vi "test_Variant to KVP.vi"(8 "error in (no error)":errorcluster) -> (0 "error out":errorcluster)   [LabVIEW 2020]
uses:
  <vilib>/addons/_JKI Toolkits/Caraya/classes/Assert/Assert Equal Value and Type_Variant.vi
  <vilib>/addons/_JKI Toolkits/Caraya/classes/Assert/Assert Not Error.vi
  <vilib>/addons/_JKI Toolkits/Caraya/classes/Test/Test.lvclass
  <vilib>/addons/_JKI Toolkits/Caraya/classes/Assert/Assert.lvclass
  _built_ppls/OpenVariant.lvlibp
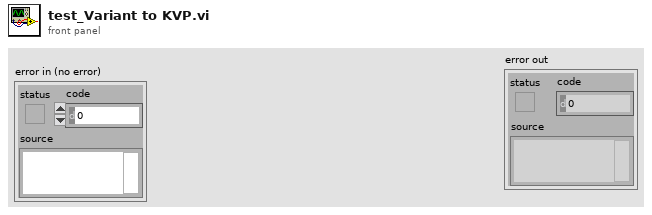
[diagram p1: front panel]
types:
  T1 = cluster{"status":bool, "source":string, "error":cluster{"status":bool, "code":i32, "source":string, "new value":i32}, "code":i32}
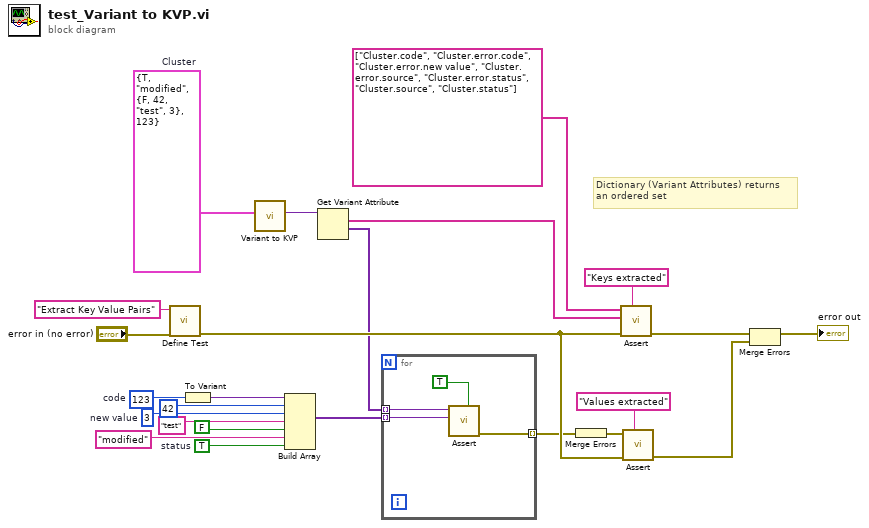
[diagram p0: block diagram]
diagram:
  w2 = TRUE  # status
  w6 = 3  # new value
  w9 = 123  # code
  w19 = T1 {"status"=TRUE, "source"="modified", "error"={"status"=FALSE, "code"=42, "source"="test", "new value"=3}, "code"=123}  # Cluster
  # "Dictionary (Variant Attributes) returns \nan ordered set"
  n1 = call <vilib>:"Define Test.vi"("error in (no error)"="error in (no error)", "Label (VI Title)"="Extract Key Value Pairs") -> ("error out"=w13:errorcluster)  [unwired: 8 in, 1 out]
  n2 = To Variant(anything=w9) -> (Variant=w8:variant)
  n3 = call "Variant to KVP.vi"("Variant"=w19) -> ("KVP Dictionary"=w18:variant)  [unwired: 10 in]
  n4 = Build Array(w8, 42 ("code"), w6, "test" ("source"), FALSE ("status"), "modified" ("source"), w2) -> (w1:variant[])
  n5 = Get Variant Attribute(Variant=w18) -> (names=w16:string[], values=w11:variant[])  [unwired: 3 in, 2 out]
  n6 = for {
    tunnel: [w28] -> w12 mode=indexing
    tunnel: w11 -> [w26] mode=indexing
    tunnel: w1 -> [w25] mode=indexing
    n7 = call-poly <vilib>:"Assert.vi"("Assert Only? (F)"=TRUE, "Y"=w25, "X"=w26) -> ("error out"=w28:errorcluster)  [unwired: 7 in, 1 out]
  }
  n8 = Merge Errors(w12) -> (w10:errorcluster)
  n9 = call-poly <vilib>:"Assert.vi"("Label"="Keys extracted" ("Label (VI Title)"), "error in (no error)"=w13, "Y"=w16, "X"=string[] ["Cluster.code", "Cluster.error.code", "Cluster.error.new value", "Cluster.error.source", "Cluster.error.status", "Cluster.source", "Cluster.status"] ("names")) -> ("error out"=w21:errorcluster)  [unwired: 6 in, 1 out]
  n10 = call-poly <vilib>:"Assert.vi"("Label"="Values extracted" ("Label (VI Title)"), "error in (no error)"=w13, "Not Error?"=w10) -> ("error out"=w14:errorcluster)  [unwired: 7 in, 1 out]
  n11 = Merge Errors(w21, w14) -> (→"error out":errorcluster)
